vi "Hatch Pannel State Machine.vi"() -> (0 "Open":bool, 3 "Extend":bool)   [LabVIEW 2018]
uses:
  SubSystems/Hatch Panel Intake/Hatch Panel Intake Global.vi
panel:
  in  "Numeric":dbl
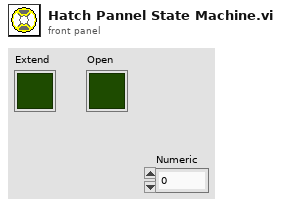
[diagram p1: front panel]
types:
  T1 = enum16{"In + Closed", "Extending + Closed", "Out + Closed", "Out + Opening", "Out + Open", "Retracting + Open", "In + Open"}
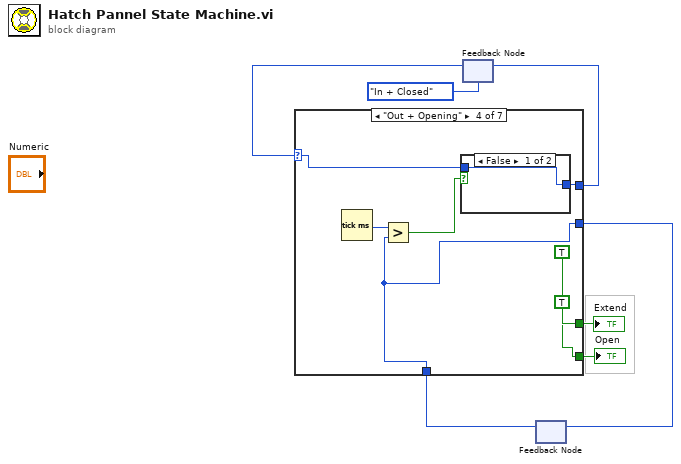
[diagram p0: block diagram]
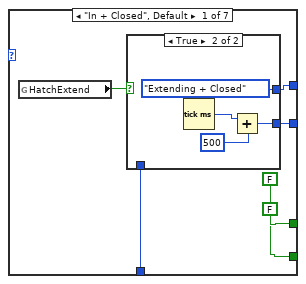
[diagram p2: hidden frame]
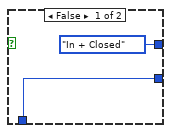
[diagram p3: hidden frame]
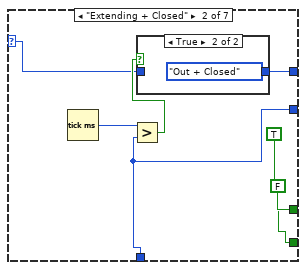
[diagram p4: hidden frame]
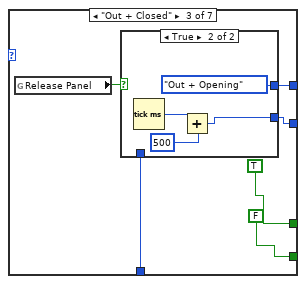
[diagram p6: hidden frame]
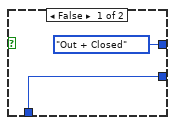
[diagram p7: hidden frame]
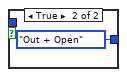
[diagram p8: hidden frame]
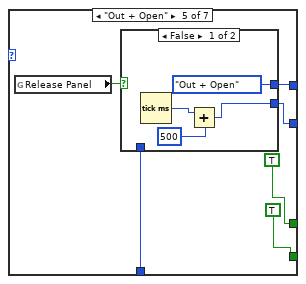
[diagram p9: hidden frame]
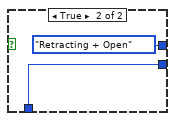
[diagram p10: hidden frame]
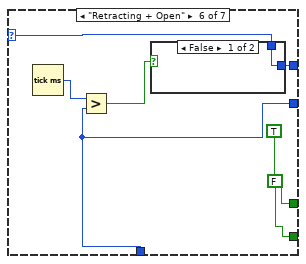
[diagram p11: hidden frame]
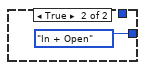
[diagram p12: hidden frame]
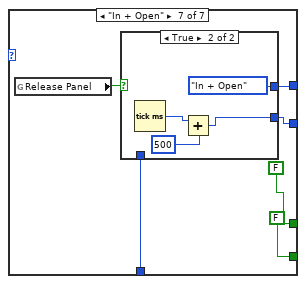
[diagram p13: hidden frame]
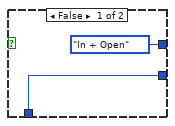
[diagram p14: hidden frame]
diagram:
  n1 = feedback #1(T1."In + Closed" ("Hatch Pannel State")) -> (w6:T1)
  n2 = feedback #2() -> (w1:u32)  [unwired: 1 in]
  n3 = case shown="\"Out + Opening\"" w6 {
    selector: w6 -> [_ w21 _ w42 _ w65 _]
    tunnel: [w13 w24 w31 w45 w54 w66 w73] -> w7
    tunnel: [FALSE TRUE TRUE TRUE TRUE TRUE FALSE] -> w4
    tunnel: [FALSE FALSE FALSE TRUE TRUE FALSE FALSE] -> w3
    tunnel: [w9 w20 w30 w41 w51 w62 w72] -> w2
    tunnel: w1 -> [w8 w20 w29 w41 w50 w62 w71]
    frame "In + Closed", Default {
      n4 = global read "Hatch Panel Intake Global.vi" "HatchExtend"() -> (w12:bool)
      n5 = case shown="True" w12 {
        tunnel: [T1."In + Closed" ("Hatch Pannel State") T1."Extending + Closed" ("Hatch Pannel State")] -> w13
        tunnel: [w14 w16] -> w9
        tunnel: w8 -> [w14 _]
        frame False {
        }
        frame True {
          n6 = Tick Count (ms)() -> (millisecond timer value=w18:u32)
          n7 = Add(x=w18, y=u32 500) -> (x+y=w16:u32)
        }
      }
    }
    frame "Extending + Closed" {
      n8 = Tick Count (ms)() -> (millisecond timer value=w23:u32)
      n9 = Greater?(x=w23, y=w20) -> (0:w22:bool)
      n10 = case shown="True" w22 {
        tunnel: [w27 T1."Out + Closed" ("Hatch Pannel State")] -> w24
        tunnel: w21 -> [w27 _]
        frame False {
        }
        frame True {
        }
      }
    }
    frame "Out + Closed" {
      n11 = global read "Hatch Panel Intake Global.vi" "Release Panel"() -> (w34:bool)
      n12 = case shown="True" w34 {
        tunnel: [T1."Out + Closed" ("Hatch Pannel State") T1."Out + Opening" ("Hatch Pannel State")] -> w31
        tunnel: [w35 w37] -> w30
        tunnel: w29 -> [w35 _]
        frame False {
        }
        frame True {
          n13 = Tick Count (ms)() -> (millisecond timer value=w39:u32)
          n14 = Add(x=w39, y=u32 500) -> (x+y=w37:u32)
        }
      }
    }
    frame "Out + Opening" {
      n15 = Tick Count (ms)() -> (millisecond timer value=w44:u32)
      n16 = Greater?(x=w44, y=w41) -> (0:w43:bool)
      n17 = case shown="False" w43 {
        tunnel: [w48 T1."Out + Open" ("Hatch Pannel State")] -> w45
        tunnel: w42 -> [w48 _]
        frame False {
        }
        frame True {
        }
      }
    }
    frame "Out + Open" {
      n18 = global read "Hatch Panel Intake Global.vi" "Release Panel"() -> (w55:bool)
      n19 = case shown="False" w55 {
        tunnel: [T1."Out + Open" ("Hatch Pannel State") T1."Retracting + Open" ("Hatch Pannel State")] -> w54
        tunnel: [w56 w60] -> w51
        tunnel: w50 -> [_ w60]
        frame False {
          n20 = Tick Count (ms)() -> (millisecond timer value=w58:u32)
          n21 = Add(x=w58, y=u32 500) -> (x+y=w56:u32)
        }
        frame True {
        }
      }
    }
    frame "Retracting + Open" {
      n22 = Tick Count (ms)() -> (millisecond timer value=w64:u32)
      n23 = Greater?(x=w64, y=w62) -> (0:w63:bool)
      n24 = case shown="False" w63 {
        tunnel: [w69 T1."In + Open" ("Hatch Pannel State")] -> w66
        tunnel: w65 -> [w69 _]
        frame False {
        }
        frame True {
        }
      }
    }
    frame "In + Open" {
      n25 = global read "Hatch Panel Intake Global.vi" "Release Panel"() -> (w76:bool)
      n26 = case shown="True" w76 {
        tunnel: [T1."In + Open" ("Hatch Pannel State") T1."In + Open" ("Hatch Pannel State")] -> w73
        tunnel: [w77 w79] -> w72
        tunnel: w71 -> [w77 _]
        frame False {
        }
        frame True {
          n27 = Tick Count (ms)() -> (millisecond timer value=w81:u32)
          n28 = Add(x=w81, y=u32 500) -> (x+y=w79:u32)
        }
      }
    }
  }
  "Open" <- w3
  "Extend" <- w4
  n29 = feedback-in #1(w7) -> ()
  n30 = feedback-in #2(w2) -> ()
